vi "Project XML Editor.vi"() -> ()   [LabVIEW 2018, in ".LVLIBP CD XML Updater.lvlib" / "Project XML Editor.lvclass"]
uses:
  Project XML Editor.lvclass
  TypeDefs/Dependency Parameters.ctl
  Project XML Editor.lvclass/Project XML Editor.ctl
panel:
  out "XML Path":path
  out "Common Doc Dir":string
  out "CD Name":string
  out "Array":T1[](array[typedef])
  out "error out":errorcluster
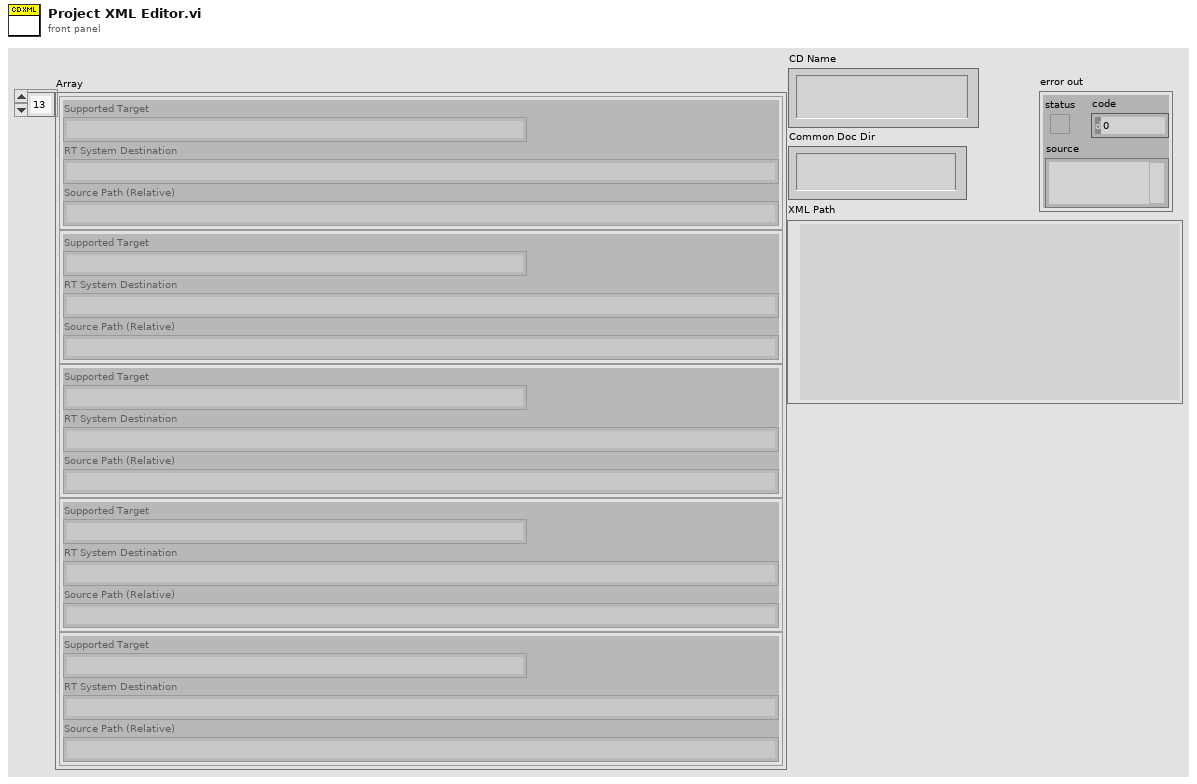
[diagram p1: front panel]
types:
  T1 = typedef ".LVLIBP CD XML Updater.lvlib/Project XML Editor.lvclass/Dependency Parameters.ctl" = cluster{"Supported Target":string, "RT System Destination":string, "Source Path (Relative)":string}
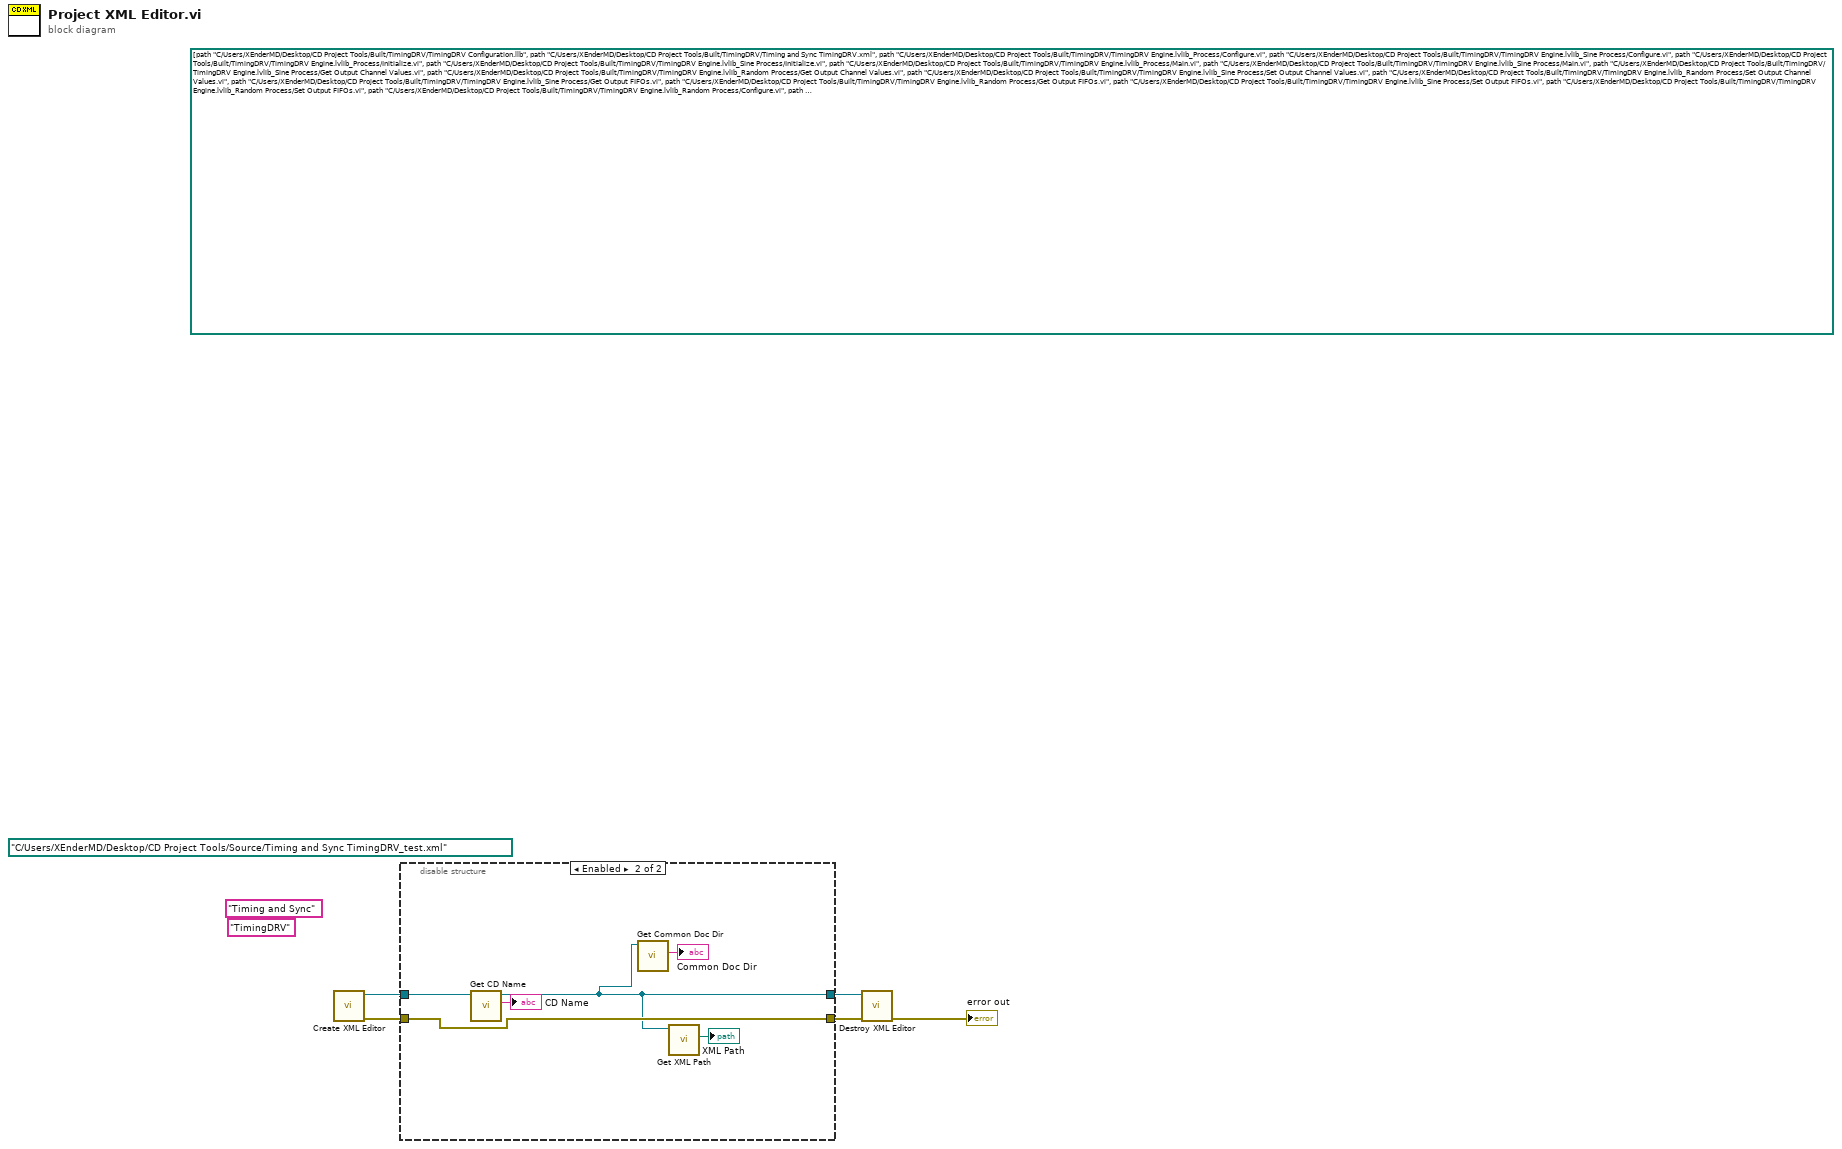
[diagram p0: block diagram]
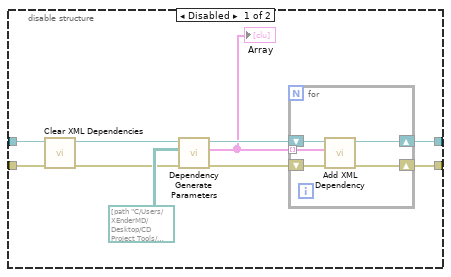
[diagram p2: hidden frame]
diagram:
  (unwired) "Timing and Sync" ("Common Doc Dir")
  (unwired) "TimingDRV" ("CD Name")
  (unwired) path "C:/Users/XEnderMD/Desktop/CD Project Tools/Source/Timing and Sync TimingDRV_test.xml" ("XML Path")
  (unwired) path[][] [[path "C:/Users/XEnderMD/Desktop/CD Project Tools/Built/TimingDRV/TimingDRV Configuration.llb", path "C:/Users/XEnderMD/Desktop/CD Project Tools/Built/TimingDRV/Timing and Sync TimingDRV.xml", path "C:/Users/XEnderMD/Desktop/CD Project Tools/Built/TimingDRV/TimingDRV Engine.lvlib_Process/Configure.vi", path "C:/Users/XEnderMD/Desktop/CD Project Tools/Built/TimingDRV/TimingDRV Engine.lvlib_Sine Process/Configure.vi", path "C:/Users/XEnderMD/Desktop/CD Project Tools/Built/TimingDRV/TimingDRV Engine.lvlib_Process/Initialize.vi", path "C:/Users/XEnderMD/Desktop/CD Project Tools/Built/TimingDRV/TimingDRV Engine.lvlib_Sine Process/Initialize.vi", path "C:/Users/XEnderMD/Desktop/CD Project Tools/Built/TimingDRV/TimingDRV Engine.lvlib_Process/Main.vi", path "C:/Users/XEnderMD/Desktop/CD Project Tools/Built/TimingDRV/TimingDRV Engine.lvlib_Sine Process/Main.vi", path "C:/Users/XEnderMD/Desktop/CD Project Tools/Built/TimingDRV/TimingDRV Engine.lvlib_Sine Process/Get Output Channel Values.vi", path "C:/Users/XEnderMD/Desktop/CD Project Tools/Built/TimingDRV/TimingDRV Engine.lvlib_Random Process/Get Output Channel Values.vi", path "C:/Users/XEnderMD/Desktop/CD Project Tools/Built/TimingDRV/TimingDRV Engine.lvlib_Sine Process/Set Output Channel Values.vi", path "C:/Users/XEnderMD/Desktop/CD Project Tools/Built/TimingDRV/TimingDRV Engine.lvlib_Random Process/Set Output Channel Values.vi", path "C:/Users/XEnderMD/Desktop/CD Project Tools/Built/TimingDRV/TimingDRV Engine.lvlib_Sine Process/Get Output FIFOs.vi", path "C:/Users/XEnderMD/Desktop/CD Project Tools/Built/TimingDRV/TimingDRV Engine.lvlib_Random Process/Get Output FIFOs.vi", path "C:/Users/XEnderMD/Desktop/CD Project Tools/Built/TimingDRV/TimingDRV Engine.lvlib_Sine Process/Set Output FIFOs.vi", path "C:/Users/XEnderMD/Desktop/CD Project Tools/Built/TimingDRV/TimingDRV Engine.lvlib_Random Process/Set Output FIFOs.vi", path "C:/Users/XEnderMD/Desktop/CD Project Tools/Built/TimingDRV/TimingDRV Engine.lvlib_Random Process/Configure.vi", path "C:/Users/XEnderMD/Desktop/CD Project Tools/Built/TimingDRV/TimingDRV Engine.lvlib_Random Process/Initialize.vi", path "C:/Users/XEnderMD/Desktop/CD Project Tools/Built/TimingDRV/TimingDRV Engine.lvlib_Sine Process/Initialize Output Channel Values.vi", path "C:/Users/XEnderMD/Desktop/CD Project Tools/Built/TimingDRV/TimingDRV Engine.lvlib_Random Process/Initialize Output Channel Values.vi", path "C:/Users/XEnderMD/Desktop/CD Project Tools/Built/TimingDRV/TimingDRV Engine.lvlib_Random Process/Main.vi", path "C:/Users/XEnderMD/Desktop/CD Project Tools/Built/TimingDRV/TimingDRV Engine.lvlib_Sine Process/Update Channel Value.vi", path "C:/Users/XEnderMD/Desktop/CD Project Tools/Built/TimingDRV/TimingDRV Engine.lvlib_Random Process/Update Channel Value.vi", path "", path "", path "", path "", path "", path "", path "", path "", path "", path "", path "", path "", path "", path "", path "", path "", path ""], [path "C:/Users/XEnderMD/Desktop/CD Project Tools/Built/TimingDRV/Windows/TimingDRV Engine Windows.llb", path "C:/Users/XEnderMD/Desktop/CD Project Tools/Built/TimingDRV/Windows/TimingDRV Engine.lvlib_Assembler/Main.vi", path "C:/Users/XEnderMD/Desktop/CD Project Tools/Built/TimingDRV/Windows/TimingDRV Engine.lvlib_Input Process/Main.vi", path "C:/Users/XEnderMD/Desktop/CD Project Tools/Built/TimingDRV/Windows/TimingDRV Engine.lvlib_Output Process/Initialize Output Channel Values.vi", path "C:/Users/XEnderMD/Desktop/CD Project Tools/Built/TimingDRV/Windows/TimingDRV Engine.lvlib_Sine Process/Initialize Output Channel Values.vi", path "C:/Users/XEnderMD/Desktop/CD Project Tools/Built/TimingDRV/Windows/TimingDRV Engine.lvlib_Output Process/Update Channel Value.vi", path "C:/Users/XEnderMD/Desktop/CD Project Tools/Built/TimingDRV/Windows/TimingDRV Engine.lvlib_Sine Process/Update Channel Value.vi", path "C:/Users/XEnderMD/Desktop/CD Project Tools/Built/TimingDRV/Windows/TimingDRV Engine.lvlib_Random Process/Initialize Output Channel Values.vi", path "C:/Users/XEnderMD/Desktop/CD Project Tools/Built/TimingDRV/Windows/TimingDRV Engine.lvlib_Random Process/Update Channel Value.vi", path "C:/Users/XEnderMD/Desktop/CD Project Tools/Built/TimingDRV/Windows/TimingDRV Engine.lvlib_Assembler/Configure.vi", path "C:/Users/XEnderMD/Desktop/CD Project Tools/Built/TimingDRV/Windows/TimingDRV Engine.lvlib_Output Process/Configure.vi", path "C:/Users/XEnderMD/Desktop/CD Project Tools/Built/TimingDRV/Windows/TimingDRV Engine.lvlib_Assembler/Initialize.vi", path "C:/Users/XEnderMD/Desktop/CD Project Tools/Built/TimingDRV/Windows/TimingDRV Engine.lvlib_Output Process/Initialize.vi", path "C:/Users/XEnderMD/Desktop/CD Project Tools/Built/TimingDRV/Windows/TimingDRV Engine.lvlib_Output Process/Main.vi", path "C:/Users/XEnderMD/Desktop/CD Project Tools/Built/TimingDRV/Windows/TimingDRV Engine.lvlib_Output Process/Get Output Channel Values.vi", path "C:/Users/XEnderMD/Desktop/CD Project Tools/Built/TimingDRV/Windows/TimingDRV Engine.lvlib_Sine Process/Get Output Channel Values.vi", path "C:/Users/XEnderMD/Desktop/CD Project Tools/Built/TimingDRV/Windows/TimingDRV Engine.lvlib_Output Process/Set Output Channel Values.vi", path "C:/Users/XEnderMD/Desktop/CD Project Tools/Built/TimingDRV/Windows/TimingDRV Engine.lvlib_Sine Process/Set Output Channel Values.vi", path "C:/Users/XEnderMD/Desktop/CD Project Tools/Built/TimingDRV/Windows/TimingDRV Engine.lvlib_Output Process/Get Output FIFOs.vi", path "C:/Users/XEnderMD/Desktop/CD Project Tools/Built/TimingDRV/Windows/TimingDRV Engine.lvlib_Sine Process/Get Output FIFOs.vi", path "C:/Users/XEnderMD/Desktop/CD Project Tools/Built/TimingDRV/Windows/TimingDRV Engine.lvlib_Output Process/Set Output FIFOs.vi", path "C:/Users/XEnderMD/Desktop/CD Project Tools/Built/TimingDRV/Windows/TimingDRV Engine.lvlib_Sine Process/Set Output FIFOs.vi", path "C:/Users/XEnderMD/Desktop/CD Project Tools/Built/TimingDRV/Windows/TimingDRV Engine.lvlib_Sine Process/Configure.vi", path "C:/Users/XEnderMD/Desktop/CD Project Tools/Built/TimingDRV/Windows/TimingDRV Engine.lvlib_Sine Process/Initialize.vi", path "C:/Users/XEnderMD/Desktop/CD Project Tools/Built/TimingDRV/Windows/TimingDRV Engine.lvlib_Sine Process/Main.vi", path "C:/Users/XEnderMD/Desktop/CD Project Tools/Built/TimingDRV/Windows/TimingDRV Engine.lvlib_Random Process/Get Output Channel Values.vi", path "C:/Users/XEnderMD/Desktop/CD Project Tools/Built/TimingDRV/Windows/TimingDRV Engine.lvlib_Random Process/Set Output Channel Values.vi", path "C:/Users/XEnderMD/Desktop/CD Project Tools/Built/TimingDRV/Windows/TimingDRV Engine.lvlib_Random Process/Get Output FIFOs.vi", path "C:/Users/XEnderMD/Desktop/CD Project Tools/Built/TimingDRV/Windows/TimingDRV Engine.lvlib_Random Process/Set Output FIFOs.vi", path "C:/Users/XEnderMD/Desktop/CD Project Tools/Built/TimingDRV/Windows/TimingDRV Engine.lvlib_Random Process/Configure.vi", path "C:/Users/XEnderMD/Desktop/CD Project Tools/Built/TimingDRV/Windows/TimingDRV Engine.lvlib_Random Process/Initialize.vi", path "C:/Users/XEnderMD/Desktop/CD Project Tools/Built/TimingDRV/Windows/TimingDRV Engine.lvlib_Random Process/Main.vi", path "C:/Users/XEnderMD/Desktop/CD Project Tools/Built/TimingDRV/Windows/TimingDRV Engine.lvlib_Process/Configure.vi", path "C:/Users/XEnderMD/Desktop/CD Project Tools/Built/TimingDRV/Windows/TimingDRV Engine.lvlib_Assembler/Launcher.vi", path "C:/Users/XEnderMD/Desktop/CD Project Tools/Built/TimingDRV/Windows/TimingDRV Engine.lvlib_Process/Launcher.vi", path "C:/Users/XEnderMD/Desktop/CD Project Tools/Built/TimingDRV/Windows/TimingDRV Engine.lvlib_Process/Initialize.vi", path "C:/Users/XEnderMD/Desktop/CD Project Tools/Built/TimingDRV/Windows/TimingDRV Engine.lvlib_Process/Main.vi", path "C:/Users/XEnderMD/Desktop/CD Project Tools/Built/TimingDRV/Windows/TimingDRV Engine.lvlib_Assembler/Shutdown.vi", path "C:/Users/XEnderMD/Desktop/CD Project Tools/Built/TimingDRV/Windows/TimingDRV Engine.lvlib_Process/Shutdown.vi", path ""], [path "C:/Users/XEnderMD/Desktop/CD Project Tools/Built/TimingDRV/Pharlap/TimingDRV Engine Pharlap.llb", path "C:/Users/XEnderMD/Desktop/CD Project Tools/Built/TimingDRV/Pharlap/TimingDRV Engine.lvlib_Assembler/Main.vi", path "C:/Users/XEnderMD/Desktop/CD Project Tools/Built/TimingDRV/Pharlap/TimingDRV Engine.lvlib_Input Process/Main.vi", path "C:/Users/XEnderMD/Desktop/CD Project Tools/Built/TimingDRV/Pharlap/TimingDRV Engine.lvlib_Output Process/Initialize Output Channel Values.vi", path "C:/Users/XEnderMD/Desktop/CD Project Tools/Built/TimingDRV/Pharlap/TimingDRV Engine.lvlib_Sine Process/Initialize Output Channel Values.vi", path "C:/Users/XEnderMD/Desktop/CD Project Tools/Built/TimingDRV/Pharlap/TimingDRV Engine.lvlib_Output Process/Update Channel Value.vi", path "C:/Users/XEnderMD/Desktop/CD Project Tools/Built/TimingDRV/Pharlap/TimingDRV Engine.lvlib_Sine Process/Update Channel Value.vi", path "C:/Users/XEnderMD/Desktop/CD Project Tools/Built/TimingDRV/Pharlap/TimingDRV Engine.lvlib_Random Process/Initialize Output Channel Values.vi", path "C:/Users/XEnderMD/Desktop/CD Project Tools/Built/TimingDRV/Pharlap/TimingDRV Engine.lvlib_Random Process/Update Channel Value.vi", path "C:/Users/XEnderMD/Desktop/CD Project Tools/Built/TimingDRV/Pharlap/TimingDRV Engine.lvlib_Assembler/Configure.vi", path "C:/Users/XEnderMD/Desktop/CD Project Tools/Built/TimingDRV/Pharlap/TimingDRV Engine.lvlib_Output Process/Configure.vi", path "C:/Users/XEnderMD/Desktop/CD Project Tools/Built/TimingDRV/Pharlap/TimingDRV Engine.lvlib_Assembler/Initialize.vi", path "C:/Users/XEnderMD/Desktop/CD Project Tools/Built/TimingDRV/Pharlap/TimingDRV Engine.lvlib_Output Process/Initialize.vi", path "C:/Users/XEnderMD/Desktop/CD Project Tools/Built/TimingDRV/Pharlap/TimingDRV Engine.lvlib_Output Process/Main.vi", path "C:/Users/XEnderMD/Desktop/CD Project Tools/Built/TimingDRV/Pharlap/TimingDRV Engine.lvlib_Output Process/Get Output Channel Values.vi", path "C:/Users/XEnderMD/Desktop/CD Project Tools/Built/TimingDRV/Pharlap/TimingDRV Engine.lvlib_Sine Process/Get Output Channel Values.vi", path "C:/Users/XEnderMD/Desktop/CD Project Tools/Built/TimingDRV/Pharlap/TimingDRV Engine.lvlib_Output Process/Set Output Channel Values.vi", path "C:/Users/XEnderMD/Desktop/CD Project Tools/Built/TimingDRV/Pharlap/TimingDRV Engine.lvlib_Sine Process/Set Output Channel Values.vi", path "C:/Users/XEnderMD/Desktop/CD Project Tools/Built/TimingDRV/Pharlap/TimingDRV Engine.lvlib_Output Process/Get Output FIFOs.vi", path "C:/Users/XEnderMD/Desktop/CD Project Tools/Built/TimingDRV/Pharlap/TimingDRV Engine.lvlib_Sine Process/Get Output FIFOs.vi", path "C:/Users/XEnderMD/Desktop/CD Project Tools/Built/TimingDRV/Pharlap/TimingDRV Engine.lvlib_Output Process/Set Output FIFOs.vi", path "C:/Users/XEnderMD/Desktop/CD Project Tools/Built/TimingDRV/Pharlap/TimingDRV Engine.lvlib_Sine Process/Set Output FIFOs.vi", path "C:/Users/XEnderMD/Desktop/CD Project Tools/Built/TimingDRV/Pharlap/TimingDRV Engine.lvlib_Sine Process/Configure.vi", path "C:/Users/XEnderMD/Desktop/CD Project Tools/Built/TimingDRV/Pharlap/TimingDRV Engine.lvlib_Sine Process/Initialize.vi", path "C:/Users/XEnderMD/Desktop/CD Project Tools/Built/TimingDRV/Pharlap/TimingDRV Engine.lvlib_Sine Process/Main.vi", path "C:/Users/XEnderMD/Desktop/CD Project Tools/Built/TimingDRV/Pharlap/TimingDRV Engine.lvlib_Random Process/Get Output Channel Values.vi", path "C:/Users/XEnderMD/Desktop/CD Project Tools/Built/TimingDRV/Pharlap/TimingDRV Engine.lvlib_Random Process/Set Output Channel Values.vi", path "C:/Users/XEnderMD/Desktop/CD Project Tools/Built/TimingDRV/Pharlap/TimingDRV Engine.lvlib_Random Process/Get Output FIFOs.vi", path "C:/Users/XEnderMD/Desktop/CD Project Tools/Built/TimingDRV/Pharlap/TimingDRV Engine.lvlib_Random Process/Set Output FIFOs.vi", path "C:/Users/XEnderMD/Desktop/CD Project Tools/Built/TimingDRV/Pharlap/TimingDRV Engine.lvlib_Random Process/Configure.vi", path "C:/Users/XEnderMD/Desktop/CD Project Tools/Built/TimingDRV/Pharlap/TimingDRV Engine.lvlib_Random Process/Initialize.vi", path "C:/Users/XEnderMD/Desktop/CD Project Tools/Built/TimingDRV/Pharlap/TimingDRV Engine.lvlib_Random Process/Main.vi", path "C:/Users/XEnderMD/Desktop/CD Project Tools/Built/TimingDRV/Pharlap/TimingDRV Engine.lvlib_Process/Configure.vi", path "C:/Users/XEnderMD/Desktop/CD Project Tools/Built/TimingDRV/Pharlap/TimingDRV Engine.lvlib_Assembler/Launcher.vi", path "C:/Users/XEnderMD/Desktop/CD Project Tools/Built/TimingDRV/Pharlap/TimingDRV Engine.lvlib_Process/Launcher.vi", path "C:/Users/XEnderMD/Desktop/CD Project Tools/Built/TimingDRV/Pharlap/TimingDRV Engine.lvlib_Process/Initialize.vi", path "C:/Users/XEnderMD/Desktop/CD Project Tools/Built/TimingDRV/Pharlap/TimingDRV Engine.lvlib_Process/Main.vi", path "C:/Users/XEnderMD/Desktop/CD Project Tools/Built/TimingDRV/Pharlap/TimingDRV Engine.lvlib_Assembler/Shutdown.vi", path "C:/Users/XEnderMD/Desktop/CD Project Tools/Built/TimingDRV/Pharlap/TimingDRV Engine.lvlib_Process/Shutdown.vi", path "C:/Users/XEnderMD/Desktop/CD Project Tools/Built/TimingDRV/Engine Release_depinstr.bin"], [path "C:/Users/XEnderMD/Desktop/CD Project Tools/Built/TimingDRV/VxWorks/TimingDRV Engine VxWorks.llb", path "C:/Users/XEnderMD/Desktop/CD Project Tools/Built/TimingDRV/VxWorks/TimingDRV Engine.lvlib_Assembler/Main.vi", path "C:/Users/XEnderMD/Desktop/CD Project Tools/Built/TimingDRV/VxWorks/TimingDRV Engine.lvlib_Input Process/Main.vi", path "C:/Users/XEnderMD/Desktop/CD Project Tools/Built/TimingDRV/VxWorks/TimingDRV Engine.lvlib_Output Process/Initialize Output Channel Values.vi", path "C:/Users/XEnderMD/Desktop/CD Project Tools/Built/TimingDRV/VxWorks/TimingDRV Engine.lvlib_Sine Process/Initialize Output Channel Values.vi", path "C:/Users/XEnderMD/Desktop/CD Project Tools/Built/TimingDRV/VxWorks/TimingDRV Engine.lvlib_Output Process/Update Channel Value.vi", path "C:/Users/XEnderMD/Desktop/CD Project Tools/Built/TimingDRV/VxWorks/TimingDRV Engine.lvlib_Sine Process/Update Channel Value.vi", path "C:/Users/XEnderMD/Desktop/CD Project Tools/Built/TimingDRV/VxWorks/TimingDRV Engine.lvlib_Random Process/Initialize Output Channel Values.vi", path "C:/Users/XEnderMD/Desktop/CD Project Tools/Built/TimingDRV/VxWorks/TimingDRV Engine.lvlib_Random Process/Update Channel Value.vi", path "C:/Users/XEnderMD/Desktop/CD Project Tools/Built/TimingDRV/VxWorks/TimingDRV Engine.lvlib_Assembler/Configure.vi", path "C:/Users/XEnderMD/Desktop/CD Project Tools/Built/TimingDRV/VxWorks/TimingDRV Engine.lvlib_Output Process/Configure.vi", path "C:/Users/XEnderMD/Desktop/CD Project Tools/Built/TimingDRV/VxWorks/TimingDRV Engine.lvlib_Assembler/Initialize.vi", path "C:/Users/XEnderMD/Desktop/CD Project Tools/Built/TimingDRV/VxWorks/TimingDRV Engine.lvlib_Output Process/Initialize.vi", path "C:/Users/XEnderMD/Desktop/CD Project Tools/Built/TimingDRV/VxWorks/TimingDRV Engine.lvlib_Output Process/Main.vi", path "C:/Users/XEnderMD/Desktop/CD Project Tools/Built/TimingDRV/VxWorks/TimingDRV Engine.lvlib_Output Process/Get Output Channel Values.vi", path "C:/Users/XEnderMD/Desktop/CD Project Tools/Built/TimingDRV/VxWorks/TimingDRV Engine.lvlib_Sine Process/Get Output Channel Values.vi", path "C:/Users/XEnderMD/Desktop/CD Project Tools/Built/TimingDRV/VxWorks/TimingDRV Engine.lvlib_Output Process/Set Output Channel Values.vi", path "C:/Users/XEnderMD/Desktop/CD Project Tools/Built/TimingDRV/VxWorks/TimingDRV Engine.lvlib_Sine Process/Set Output Channel Values.vi", path "C:/Users/XEnderMD/Desktop/CD Project Tools/Built/TimingDRV/VxWorks/TimingDRV Engine.lvlib_Output Process/Get Output FIFOs.vi", path "C:/Users/XEnderMD/Desktop/CD Project Tools/Built/TimingDRV/VxWorks/TimingDRV Engine.lvlib_Sine Process/Get Output FIFOs.vi", path "C:/Users/XEnderMD/Desktop/CD Project Tools/Built/TimingDRV/VxWorks/TimingDRV Engine.lvlib_Output Process/Set Output FIFOs.vi", path "C:/Users/XEnderMD/Desktop/CD Project Tools/Built/TimingDRV/VxWorks/TimingDRV Engine.lvlib_Sine Process/Set Output FIFOs.vi", path "C:/Users/XEnderMD/Desktop/CD Project Tools/Built/TimingDRV/VxWorks/TimingDRV Engine.lvlib_Sine Process/Configure.vi", path "C:/Users/XEnderMD/Desktop/CD Project Tools/Built/TimingDRV/VxWorks/TimingDRV Engine.lvlib_Sine Process/Initialize.vi", path "C:/Users/XEnderMD/Desktop/CD Project Tools/Built/TimingDRV/VxWorks/TimingDRV Engine.lvlib_Sine Process/Main.vi", path "C:/Users/XEnderMD/Desktop/CD Project Tools/Built/TimingDRV/VxWorks/TimingDRV Engine.lvlib_Random Process/Get Output Channel Values.vi", path "C:/Users/XEnderMD/Desktop/CD Project Tools/Built/TimingDRV/VxWorks/TimingDRV Engine.lvlib_Random Process/Set Output Channel Values.vi", path "C:/Users/XEnderMD/Desktop/CD Project Tools/Built/TimingDRV/VxWorks/TimingDRV Engine.lvlib_Random Process/Get Output FIFOs.vi", path "C:/Users/XEnderMD/Desktop/CD Project Tools/Built/TimingDRV/VxWorks/TimingDRV Engine.lvlib_Random Process/Set Output FIFOs.vi", path "C:/Users/XEnderMD/Desktop/CD Project Tools/Built/TimingDRV/VxWorks/TimingDRV Engine.lvlib_Random Process/Configure.vi", path "C:/Users/XEnderMD/Desktop/CD Project Tools/Built/TimingDRV/VxWorks/TimingDRV Engine.lvlib_Random Process/Initialize.vi", path "C:/Users/XEnderMD/Desktop/CD Project Tools/Built/TimingDRV/VxWorks/TimingDRV Engine.lvlib_Random Process/Main.vi", path "C:/Users/XEnderMD/Desktop/CD Project Tools/Built/TimingDRV/VxWorks/TimingDRV Engine.lvlib_Process/Configure.vi", path "C:/Users/XEnderMD/Desktop/CD Project Tools/Built/TimingDRV/VxWorks/TimingDRV Engine.lvlib_Assembler/Launcher.vi", path "C:/Users/XEnderMD/Desktop/CD Project Tools/Built/TimingDRV/VxWorks/TimingDRV Engine.lvlib_Process/Launcher.vi", path "C:/Users/XEnderMD/Desktop/CD Project Tools/Built/TimingDRV/VxWorks/TimingDRV Engine.lvlib_Process/Initialize.vi", path "C:/Users/XEnderMD/Desktop/CD Project Tools/Built/TimingDRV/VxWorks/TimingDRV Engine.lvlib_Process/Main.vi", path "C:/Users/XEnderMD/Desktop/CD Project Tools/Built/TimingDRV/VxWorks/TimingDRV Engine.lvlib_Assembler/Shutdown.vi", path "C:/Users/XEnderMD/Desktop/CD Project Tools/Built/TimingDRV/VxWorks/TimingDRV Engine.lvlib_Process/Shutdown.vi", path "C:/Users/XEnderMD/Desktop/CD Project Tools/Built/TimingDRV/Engine Release_depinstr.bin"], [path "C:/Users/XEnderMD/Desktop/CD Project Tools/Built/TimingDRV/Linux_32_ARM/TimingDRV Engine LinuxARM.llb", path "C:/Users/XEnderMD/Desktop/CD Project Tools/Built/TimingDRV/Linux_32_ARM/TimingDRV Engine.lvlib_Assembler/Main.vi", path "C:/Users/XEnderMD/Desktop/CD Project Tools/Built/TimingDRV/Linux_32_ARM/TimingDRV Engine.lvlib_Input Process/Main.vi", path "C:/Users/XEnderMD/Desktop/CD Project Tools/Built/TimingDRV/Linux_32_ARM/TimingDRV Engine.lvlib_Output Process/Initialize Output Channel Values.vi", path "C:/Users/XEnderMD/Desktop/CD Project Tools/Built/TimingDRV/Linux_32_ARM/TimingDRV Engine.lvlib_Sine Process/Initialize Output Channel Values.vi", path "C:/Users/XEnderMD/Desktop/CD Project Tools/Built/TimingDRV/Linux_32_ARM/TimingDRV Engine.lvlib_Output Process/Update Channel Value.vi", path "C:/Users/XEnderMD/Desktop/CD Project Tools/Built/TimingDRV/Linux_32_ARM/TimingDRV Engine.lvlib_Sine Process/Update Channel Value.vi", path "C:/Users/XEnderMD/Desktop/CD Project Tools/Built/TimingDRV/Linux_32_ARM/TimingDRV Engine.lvlib_Random Process/Initialize Output Channel Values.vi", path "C:/Users/XEnderMD/Desktop/CD Project Tools/Built/TimingDRV/Linux_32_ARM/TimingDRV Engine.lvlib_Random Process/Update Channel Value.vi", path "C:/Users/XEnderMD/Desktop/CD Project Tools/Built/TimingDRV/Linux_32_ARM/TimingDRV Engine.lvlib_Assembler/Configure.vi", path "C:/Users/XEnderMD/Desktop/CD Project Tools/Built/TimingDRV/Linux_32_ARM/TimingDRV Engine.lvlib_Output Process/Configure.vi", path "C:/Users/XEnderMD/Desktop/CD Project Tools/Built/TimingDRV/Linux_32_ARM/TimingDRV Engine.lvlib_Assembler/Initialize.vi", path "C:/Users/XEnderMD/Desktop/CD Project Tools/Built/TimingDRV/Linux_32_ARM/TimingDRV Engine.lvlib_Output Process/Initialize.vi", path "C:/Users/XEnderMD/Desktop/CD Project Tools/Built/TimingDRV/Linux_32_ARM/TimingDRV Engine.lvlib_Output Process/Main.vi", path "C:/Users/XEnderMD/Desktop/CD Project Tools/Built/TimingDRV/Linux_32_ARM/TimingDRV Engine.lvlib_Output Process/Get Output Channel Values.vi", path "C:/Users/XEnderMD/Desktop/CD Project Tools/Built/TimingDRV/Linux_32_ARM/TimingDRV Engine.lvlib_Sine Process/Get Output Channel Values.vi", path "C:/Users/XEnderMD/Desktop/CD Project Tools/Built/TimingDRV/Linux_32_ARM/TimingDRV Engine.lvlib_Output Process/Set Output Channel Values.vi", path "C:/Users/XEnderMD/Desktop/CD Project Tools/Built/TimingDRV/Linux_32_ARM/TimingDRV Engine.lvlib_Sine Process/Set Output Channel Values.vi", path "C:/Users/XEnderMD/Desktop/CD Project Tools/Built/TimingDRV/Linux_32_ARM/TimingDRV Engine.lvlib_Output Process/Get Output FIFOs.vi", path "C:/Users/XEnderMD/Desktop/CD Project Tools/Built/TimingDRV/Linux_32_ARM/TimingDRV Engine.lvlib_Sine Process/Get Output FIFOs.vi", path "C:/Users/XEnderMD/Desktop/CD Project Tools/Built/TimingDRV/Linux_32_ARM/TimingDRV Engine.lvlib_Output Process/Set Output FIFOs.vi", path "C:/Users/XEnderMD/Desktop/CD Project Tools/Built/TimingDRV/Linux_32_ARM/TimingDRV Engine.lvlib_Sine Process/Set Output FIFOs.vi", path "C:/Users/XEnderMD/Desktop/CD Project Tools/Built/TimingDRV/Linux_32_ARM/TimingDRV Engine.lvlib_Sine Process/Configure.vi", path "C:/Users/XEnderMD/Desktop/CD Project Tools/Built/TimingDRV/Linux_32_ARM/TimingDRV Engine.lvlib_Sine Process/Initialize.vi", path "C:/Users/XEnderMD/Desktop/CD Project Tools/Built/TimingDRV/Linux_32_ARM/TimingDRV Engine.lvlib_Sine Process/Main.vi", path "C:/Users/XEnderMD/Desktop/CD Project Tools/Built/TimingDRV/Linux_32_ARM/TimingDRV Engine.lvlib_Random Process/Get Output Channel Values.vi", path "C:/Users/XEnderMD/Desktop/CD Project Tools/Built/TimingDRV/Linux_32_ARM/TimingDRV Engine.lvlib_Random Process/Set Output Channel Values.vi", path "C:/Users/XEnderMD/Desktop/CD Project Tools/Built/TimingDRV/Linux_32_ARM/TimingDRV Engine.lvlib_Random Process/Get Output FIFOs.vi", path "C:/Users/XEnderMD/Desktop/CD Project Tools/Built/TimingDRV/Linux_32_ARM/TimingDRV Engine.lvlib_Random Process/Set Output FIFOs.vi", path "C:/Users/XEnderMD/Desktop/CD Project Tools/Built/TimingDRV/Linux_32_ARM/TimingDRV Engine.lvlib_Random Process/Configure.vi", path "C:/Users/XEnderMD/Desktop/CD Project Tools/Built/TimingDRV/Linux_32_ARM/TimingDRV Engine.lvlib_Random Process/Initialize.vi", path "C:/Users/XEnderMD/Desktop/CD Project Tools/Built/TimingDRV/Linux_32_ARM/TimingDRV Engine.lvlib_Random Process/Main.vi", path "C:/Users/XEnderMD/Desktop/CD Project Tools/Built/TimingDRV/Linux_32_ARM/TimingDRV Engine.lvlib_Process/Configure.vi", path "C:/Users/XEnderMD/Desktop/CD Project Tools/Built/TimingDRV/Linux_32_ARM/TimingDRV Engine.lvlib_Assembler/Launcher.vi", path "C:/Users/XEnderMD/Desktop/CD Project Tools/Built/TimingDRV/Linux_32_ARM/TimingDRV Engine.lvlib_Process/Launcher.vi", path "C:/Users/XEnderMD/Desktop/CD Project Tools/Built/TimingDRV/Linux_32_ARM/TimingDRV Engine.lvlib_Process/Initialize.vi", path "C:/Users/XEnderMD/Desktop/CD Project Tools/Built/TimingDRV/Linux_32_ARM/TimingDRV Engine.lvlib_Process/Main.vi", path "C:/Users/XEnderMD/Desktop/CD Project Tools/Built/TimingDRV/Linux_32_ARM/TimingDRV Engine.lvlib_Assembler/Shutdown.vi", path "C:/Users/XEnderMD/Desktop/CD Project Tools/Built/TimingDRV/Linux_32_ARM/TimingDRV Engine.lvlib_Process/Shutdown.vi", path "C:/Users/XEnderMD/Desktop/CD Project Tools/Built/TimingDRV/Engine Release_depinstr.bin"], [path "C:/Users/XEnderMD/Desktop/CD Project Tools/Built/TimingDRV/Linux_x64/TimingDRV Engine Linux64.llb", path "C:/Users/XEnderMD/Desktop/CD Project Tools/Built/TimingDRV/Linux_x64/TimingDRV Engine.lvlib_Assembler/Main.vi", path "C:/Users/XEnderMD/Desktop/CD Project Tools/Built/TimingDRV/Linux_x64/TimingDRV Engine.lvlib_Input Process/Main.vi", path "C:/Users/XEnderMD/Desktop/CD Project Tools/Built/TimingDRV/Linux_x64/TimingDRV Engine.lvlib_Output Process/Initialize Output Channel Values.vi", path "C:/Users/XEnderMD/Desktop/CD Project Tools/Built/TimingDRV/Linux_x64/TimingDRV Engine.lvlib_Sine Process/Initialize Output Channel Values.vi", path "C:/Users/XEnderMD/Desktop/CD Project Tools/Built/TimingDRV/Linux_x64/TimingDRV Engine.lvlib_Output Process/Update Channel Value.vi", path "C:/Users/XEnderMD/Desktop/CD Project Tools/Built/TimingDRV/Linux_x64/TimingDRV Engine.lvlib_Sine Process/Update Channel Value.vi", path "C:/Users/XEnderMD/Desktop/CD Project Tools/Built/TimingDRV/Linux_x64/TimingDRV Engine.lvlib_Random Process/Initialize Output Channel Values.vi", path "C:/Users/XEnderMD/Desktop/CD Project Tools/Built/TimingDRV/Linux_x64/TimingDRV Engine.lvlib_Random Process/Update Channel Value.vi", path "C:/Users/XEnderMD/Desktop/CD Project Tools/Built/TimingDRV/Linux_x64/TimingDRV Engine.lvlib_Assembler/Configure.vi", path "C:/Users/XEnderMD/Desktop/CD Project Tools/Built/TimingDRV/Linux_x64/TimingDRV Engine.lvlib_Output Process/Configure.vi", path "C:/Users/XEnderMD/Desktop/CD Project Tools/Built/TimingDRV/Linux_x64/TimingDRV Engine.lvlib_Assembler/Initialize.vi", path "C:/Users/XEnderMD/Desktop/CD Project Tools/Built/TimingDRV/Linux_x64/TimingDRV Engine.lvlib_Output Process/Initialize.vi", path "C:/Users/XEnderMD/Desktop/CD Project Tools/Built/TimingDRV/Linux_x64/TimingDRV Engine.lvlib_Output Process/Main.vi", path "C:/Users/XEnderMD/Desktop/CD Project Tools/Built/TimingDRV/Linux_x64/TimingDRV Engine.lvlib_Output Process/Get Output Channel Values.vi", path "C:/Users/XEnderMD/Desktop/CD Project Tools/Built/TimingDRV/Linux_x64/TimingDRV Engine.lvlib_Sine Process/Get Output Channel Values.vi", path "C:/Users/XEnderMD/Desktop/CD Project Tools/Built/TimingDRV/Linux_x64/TimingDRV Engine.lvlib_Output Process/Set Output Channel Values.vi", path "C:/Users/XEnderMD/Desktop/CD Project Tools/Built/TimingDRV/Linux_x64/TimingDRV Engine.lvlib_Sine Process/Set Output Channel Values.vi", path "C:/Users/XEnderMD/Desktop/CD Project Tools/Built/TimingDRV/Linux_x64/TimingDRV Engine.lvlib_Output Process/Get Output FIFOs.vi", path "C:/Users/XEnderMD/Desktop/CD Project Tools/Built/TimingDRV/Linux_x64/TimingDRV Engine.lvlib_Sine Process/Get Output FIFOs.vi", path "C:/Users/XEnderMD/Desktop/CD Project Tools/Built/TimingDRV/Linux_x64/TimingDRV Engine.lvlib_Output Process/Set Output FIFOs.vi", path "C:/Users/XEnderMD/Desktop/CD Project Tools/Built/TimingDRV/Linux_x64/TimingDRV Engine.lvlib_Sine Process/Set Output FIFOs.vi", path "C:/Users/XEnderMD/Desktop/CD Project Tools/Built/TimingDRV/Linux_x64/TimingDRV Engine.lvlib_Sine Process/Configure.vi", path "C:/Users/XEnderMD/Desktop/CD Project Tools/Built/TimingDRV/Linux_x64/TimingDRV Engine.lvlib_Sine Process/Initialize.vi", path "C:/Users/XEnderMD/Desktop/CD Project Tools/Built/TimingDRV/Linux_x64/TimingDRV Engine.lvlib_Sine Process/Main.vi", path "C:/Users/XEnderMD/Desktop/CD Project Tools/Built/TimingDRV/Linux_x64/TimingDRV Engine.lvlib_Random Process/Get Output Channel Values.vi", path "C:/Users/XEnderMD/Desktop/CD Project Tools/Built/TimingDRV/Linux_x64/TimingDRV Engine.lvlib_Random Process/Set Output Channel Values.vi", path "C:/Users/XEnderMD/Desktop/CD Project Tools/Built/TimingDRV/Linux_x64/TimingDRV Engine.lvlib_Random Process/Get Output FIFOs.vi", path "C:/Users/XEnderMD/Desktop/CD Project Tools/Built/TimingDRV/Linux_x64/TimingDRV Engine.lvlib_Random Process/Set Output FIFOs.vi", path "C:/Users/XEnderMD/Desktop/CD Project Tools/Built/TimingDRV/Linux_x64/TimingDRV Engine.lvlib_Random Process/Configure.vi", path "C:/Users/XEnderMD/Desktop/CD Project Tools/Built/TimingDRV/Linux_x64/TimingDRV Engine.lvlib_Random Process/Initialize.vi", path "C:/Users/XEnderMD/Desktop/CD Project Tools/Built/TimingDRV/Linux_x64/TimingDRV Engine.lvlib_Random Process/Main.vi", path "C:/Users/XEnderMD/Desktop/CD Project Tools/Built/TimingDRV/Linux_x64/TimingDRV Engine.lvlib_Process/Configure.vi", path "C:/Users/XEnderMD/Desktop/CD Project Tools/Built/TimingDRV/Linux_x64/TimingDRV Engine.lvlib_Assembler/Launcher.vi", path "C:/Users/XEnderMD/Desktop/CD Project Tools/Built/TimingDRV/Linux_x64/TimingDRV Engine.lvlib_Process/Launcher.vi", path "C:/Users/XEnderMD/Desktop/CD Project Tools/Built/TimingDRV/Linux_x64/TimingDRV Engine.lvlib_Process/Initialize.vi", path "C:/Users/XEnderMD/Desktop/CD Project Tools/Built/TimingDRV/Linux_x64/TimingDRV Engine.lvlib_Process/Main.vi", path "C:/Users/XEnderMD/Desktop/CD Project Tools/Built/TimingDRV/Linux_x64/TimingDRV Engine.lvlib_Assembler/Shutdown.vi", path "C:/Users/XEnderMD/Desktop/CD Project Tools/Built/TimingDRV/Linux_x64/TimingDRV Engine.lvlib_Process/Shutdown.vi", path "C:/Users/XEnderMD/Desktop/CD Project Tools/Built/TimingDRV/Engine Release_depinstr.bin"]] ("Generated files 2")
  n1 = call "Create XML Editor.vi"() -> ("error out"=w1:errorcluster, "Project XML Editor out"=w2:refnum<class "Project XML Editor.lvclass">)  [unwired: 10 in]
  n2 = disable-structure shown="Enabled" {
    disable-tunnel: [w14 w22] -> w4
    disable-tunnel: [w13 w25] -> w3
    disable-tunnel: w2 -> [w12 w26]
    disable-tunnel: w1 -> [w11 w25]
    frame Disabled {
      n3 = call "Clear XML Dependencies.vi"("error in (no error)"=w11, "Project XML Editor in"=w12) -> ("error out"=w10:errorcluster, "Project XML Editor out"=w9:refnum<class "Project XML Editor.lvclass">)  [unwired: 8 in]
      n4 = call "Dependency Generate Parameters.vi"("error in (no error)"=w10, "Generated files in"=path[][] [[path "C:/Users/XEnderMD/Desktop/CD Project Tools/Built/TimingDRV/TimingDRV Configuration.llb", path "C:/Users/XEnderMD/Desktop/CD Project Tools/Built/TimingDRV/Timing and Sync TimingDRV.xml", path "C:/Users/XEnderMD/Desktop/CD Project Tools/Built/TimingDRV/TimingDRV Engine.lvlib_Process/Configure.vi", path "C:/Users/XEnderMD/Desktop/CD Project Tools/Built/TimingDRV/TimingDRV Engine.lvlib_Sine Process/Configure.vi", path "C:/Users/XEnderMD/Desktop/CD Project Tools/Built/TimingDRV/TimingDRV Engine.lvlib_Process/Initialize.vi", path "C:/Users/XEnderMD/Desktop/CD Project Tools/Built/TimingDRV/TimingDRV Engine.lvlib_Sine Process/Initialize.vi", path "C:/Users/XEnderMD/Desktop/CD Project Tools/Built/TimingDRV/TimingDRV Engine.lvlib_Process/Main.vi", path "C:/Users/XEnderMD/Desktop/CD Project Tools/Built/TimingDRV/TimingDRV Engine.lvlib_Sine Process/Main.vi", path "C:/Users/XEnderMD/Desktop/CD Project Tools/Built/TimingDRV/TimingDRV Engine.lvlib_Sine Process/Get Output Channel Values.vi", path "C:/Users/XEnderMD/Desktop/CD Project Tools/Built/TimingDRV/TimingDRV Engine.lvlib_Random Process/Get Output Channel Values.vi", path "C:/Users/XEnderMD/Desktop/CD Project Tools/Built/TimingDRV/TimingDRV Engine.lvlib_Sine Process/Set Output Channel Values.vi", path "C:/Users/XEnderMD/Desktop/CD Project Tools/Built/TimingDRV/TimingDRV Engine.lvlib_Random Process/Set Output Channel Values.vi", path "C:/Users/XEnderMD/Desktop/CD Project Tools/Built/TimingDRV/TimingDRV Engine.lvlib_Sine Process/Get Output FIFOs.vi", path "C:/Users/XEnderMD/Desktop/CD Project Tools/Built/TimingDRV/TimingDRV Engine.lvlib_Random Process/Get Output FIFOs.vi", path "C:/Users/XEnderMD/Desktop/CD Project Tools/Built/TimingDRV/TimingDRV Engine.lvlib_Sine Process/Set Output FIFOs.vi", path "C:/Users/XEnderMD/Desktop/CD Project Tools/Built/TimingDRV/TimingDRV Engine.lvlib_Random Process/Set Output FIFOs.vi", path "C:/Users/XEnderMD/Desktop/CD Project Tools/Built/TimingDRV/TimingDRV Engine.lvlib_Random Process/Configure.vi", path "C:/Users/XEnderMD/Desktop/CD Project Tools/Built/TimingDRV/TimingDRV Engine.lvlib_Random Process/Initialize.vi", path "C:/Users/XEnderMD/Desktop/CD Project Tools/Built/TimingDRV/TimingDRV Engine.lvlib_Sine Process/Initialize Output Channel Values.vi", path "C:/Users/XEnderMD/Desktop/CD Project Tools/Built/TimingDRV/TimingDRV Engine.lvlib_Random Process/Initialize Output Channel Values.vi", path "C:/Users/XEnderMD/Desktop/CD Project Tools/Built/TimingDRV/TimingDRV Engine.lvlib_Random Process/Main.vi", path "C:/Users/XEnderMD/Desktop/CD Project Tools/Built/TimingDRV/TimingDRV Engine.lvlib_Sine Process/Update Channel Value.vi", path "C:/Users/XEnderMD/Desktop/CD Project Tools/Built/TimingDRV/TimingDRV Engine.lvlib_Random Process/Update Channel Value.vi", path "", path "", path "", path "", path "", path "", path "", path "", path "", path "", path "", path "", path "", path "", path "", path "", path ""], [path "C:/Users/XEnderMD/Desktop/CD Project Tools/Built/TimingDRV/Windows/TimingDRV Engine Windows.llb", path "C:/Users/XEnderMD/Desktop/CD Project Tools/Built/TimingDRV/Windows/TimingDRV Engine.lvlib_Assembler/Main.vi", path "C:/Users/XEnderMD/Desktop/CD Project Tools/Built/TimingDRV/Windows/TimingDRV Engine.lvlib_Input Process/Main.vi", path "C:/Users/XEnderMD/Desktop/CD Project Tools/Built/TimingDRV/Windows/TimingDRV Engine.lvlib_Output Process/Initialize Output Channel Values.vi", path "C:/Users/XEnderMD/Desktop/CD Project Tools/Built/TimingDRV/Windows/TimingDRV Engine.lvlib_Sine Process/Initialize Output Channel Values.vi", path "C:/Users/XEnderMD/Desktop/CD Project Tools/Built/TimingDRV/Windows/TimingDRV Engine.lvlib_Output Process/Update Channel Value.vi", path "C:/Users/XEnderMD/Desktop/CD Project Tools/Built/TimingDRV/Windows/TimingDRV Engine.lvlib_Sine Process/Update Channel Value.vi", path "C:/Users/XEnderMD/Desktop/CD Project Tools/Built/TimingDRV/Windows/TimingDRV Engine.lvlib_Random Process/Initialize Output Channel Values.vi", path "C:/Users/XEnderMD/Desktop/CD Project Tools/Built/TimingDRV/Windows/TimingDRV Engine.lvlib_Random Process/Update Channel Value.vi", path "C:/Users/XEnderMD/Desktop/CD Project Tools/Built/TimingDRV/Windows/TimingDRV Engine.lvlib_Assembler/Configure.vi", path "C:/Users/XEnderMD/Desktop/CD Project Tools/Built/TimingDRV/Windows/TimingDRV Engine.lvlib_Output Process/Configure.vi", path "C:/Users/XEnderMD/Desktop/CD Project Tools/Built/TimingDRV/Windows/TimingDRV Engine.lvlib_Assembler/Initialize.vi", path "C:/Users/XEnderMD/Desktop/CD Project Tools/Built/TimingDRV/Windows/TimingDRV Engine.lvlib_Output Process/Initialize.vi", path "C:/Users/XEnderMD/Desktop/CD Project Tools/Built/TimingDRV/Windows/TimingDRV Engine.lvlib_Output Process/Main.vi", path "C:/Users/XEnderMD/Desktop/CD Project Tools/Built/TimingDRV/Windows/TimingDRV Engine.lvlib_Output Process/Get Output Channel Values.vi", path "C:/Users/XEnderMD/Desktop/CD Project Tools/Built/TimingDRV/Windows/TimingDRV Engine.lvlib_Sine Process/Get Output Channel Values.vi", path "C:/Users/XEnderMD/Desktop/CD Project Tools/Built/TimingDRV/Windows/TimingDRV Engine.lvlib_Output Process/Set Output Channel Values.vi", path "C:/Users/XEnderMD/Desktop/CD Project Tools/Built/TimingDRV/Windows/TimingDRV Engine.lvlib_Sine Process/Set Output Channel Values.vi", path "C:/Users/XEnderMD/Desktop/CD Project Tools/Built/TimingDRV/Windows/TimingDRV Engine.lvlib_Output Process/Get Output FIFOs.vi", path "C:/Users/XEnderMD/Desktop/CD Project Tools/Built/TimingDRV/Windows/TimingDRV Engine.lvlib_Sine Process/Get Output FIFOs.vi", path "C:/Users/XEnderMD/Desktop/CD Project Tools/Built/TimingDRV/Windows/TimingDRV Engine.lvlib_Output Process/Set Output FIFOs.vi", path "C:/Users/XEnderMD/Desktop/CD Project Tools/Built/TimingDRV/Windows/TimingDRV Engine.lvlib_Sine Process/Set Output FIFOs.vi", path "C:/Users/XEnderMD/Desktop/CD Project Tools/Built/TimingDRV/Windows/TimingDRV Engine.lvlib_Sine Process/Configure.vi", path "C:/Users/XEnderMD/Desktop/CD Project Tools/Built/TimingDRV/Windows/TimingDRV Engine.lvlib_Sine Process/Initialize.vi", path "C:/Users/XEnderMD/Desktop/CD Project Tools/Built/TimingDRV/Windows/TimingDRV Engine.lvlib_Sine Process/Main.vi", path "C:/Users/XEnderMD/Desktop/CD Project Tools/Built/TimingDRV/Windows/TimingDRV Engine.lvlib_Random Process/Get Output Channel Values.vi", path "C:/Users/XEnderMD/Desktop/CD Project Tools/Built/TimingDRV/Windows/TimingDRV Engine.lvlib_Random Process/Set Output Channel Values.vi", path "C:/Users/XEnderMD/Desktop/CD Project Tools/Built/TimingDRV/Windows/TimingDRV Engine.lvlib_Random Process/Get Output FIFOs.vi", path "C:/Users/XEnderMD/Desktop/CD Project Tools/Built/TimingDRV/Windows/TimingDRV Engine.lvlib_Random Process/Set Output FIFOs.vi", path "C:/Users/XEnderMD/Desktop/CD Project Tools/Built/TimingDRV/Windows/TimingDRV Engine.lvlib_Random Process/Configure.vi", path "C:/Users/XEnderMD/Desktop/CD Project Tools/Built/TimingDRV/Windows/TimingDRV Engine.lvlib_Random Process/Initialize.vi", path "C:/Users/XEnderMD/Desktop/CD Project Tools/Built/TimingDRV/Windows/TimingDRV Engine.lvlib_Random Process/Main.vi", path "C:/Users/XEnderMD/Desktop/CD Project Tools/Built/TimingDRV/Windows/TimingDRV Engine.lvlib_Process/Configure.vi", path "C:/Users/XEnderMD/Desktop/CD Project Tools/Built/TimingDRV/Windows/TimingDRV Engine.lvlib_Assembler/Launcher.vi", path "C:/Users/XEnderMD/Desktop/CD Project Tools/Built/TimingDRV/Windows/TimingDRV Engine.lvlib_Process/Launcher.vi", path "C:/Users/XEnderMD/Desktop/CD Project Tools/Built/TimingDRV/Windows/TimingDRV Engine.lvlib_Process/Initialize.vi", path "C:/Users/XEnderMD/Desktop/CD Project Tools/Built/TimingDRV/Windows/TimingDRV Engine.lvlib_Process/Main.vi", path "C:/Users/XEnderMD/Desktop/CD Project Tools/Built/TimingDRV/Windows/TimingDRV Engine.lvlib_Assembler/Shutdown.vi", path "C:/Users/XEnderMD/Desktop/CD Project Tools/Built/TimingDRV/Windows/TimingDRV Engine.lvlib_Process/Shutdown.vi", path ""], [path "C:/Users/XEnderMD/Desktop/CD Project Tools/Built/TimingDRV/Pharlap/TimingDRV Engine Pharlap.llb", path "C:/Users/XEnderMD/Desktop/CD Project Tools/Built/TimingDRV/Pharlap/TimingDRV Engine.lvlib_Assembler/Main.vi", path "C:/Users/XEnderMD/Desktop/CD Project Tools/Built/TimingDRV/Pharlap/TimingDRV Engine.lvlib_Input Process/Main.vi", path "C:/Users/XEnderMD/Desktop/CD Project Tools/Built/TimingDRV/Pharlap/TimingDRV Engine.lvlib_Output Process/Initialize Output Channel Values.vi", path "C:/Users/XEnderMD/Desktop/CD Project Tools/Built/TimingDRV/Pharlap/TimingDRV Engine.lvlib_Sine Process/Initialize Output Channel Values.vi", path "C:/Users/XEnderMD/Desktop/CD Project Tools/Built/TimingDRV/Pharlap/TimingDRV Engine.lvlib_Output Process/Update Channel Value.vi", path "C:/Users/XEnderMD/Desktop/CD Project Tools/Built/TimingDRV/Pharlap/TimingDRV Engine.lvlib_Sine Process/Update Channel Value.vi", path "C:/Users/XEnderMD/Desktop/CD Project Tools/Built/TimingDRV/Pharlap/TimingDRV Engine.lvlib_Random Process/Initialize Output Channel Values.vi", path "C:/Users/XEnderMD/Desktop/CD Project Tools/Built/TimingDRV/Pharlap/TimingDRV Engine.lvlib_Random Process/Update Channel Value.vi", path "C:/Users/XEnderMD/Desktop/CD Project Tools/Built/TimingDRV/Pharlap/TimingDRV Engine.lvlib_Assembler/Configure.vi", path "C:/Users/XEnderMD/Desktop/CD Project Tools/Built/TimingDRV/Pharlap/TimingDRV Engine.lvlib_Output Process/Configure.vi", path "C:/Users/XEnderMD/Desktop/CD Project Tools/Built/TimingDRV/Pharlap/TimingDRV Engine.lvlib_Assembler/Initialize.vi", path "C:/Users/XEnderMD/Desktop/CD Project Tools/Built/TimingDRV/Pharlap/TimingDRV Engine.lvlib_Output Process/Initialize.vi", path "C:/Users/XEnderMD/Desktop/CD Project Tools/Built/TimingDRV/Pharlap/TimingDRV Engine.lvlib_Output Process/Main.vi", path "C:/Users/XEnderMD/Desktop/CD Project Tools/Built/TimingDRV/Pharlap/TimingDRV Engine.lvlib_Output Process/Get Output Channel Values.vi", path "C:/Users/XEnderMD/Desktop/CD Project Tools/Built/TimingDRV/Pharlap/TimingDRV Engine.lvlib_Sine Process/Get Output Channel Values.vi", path "C:/Users/XEnderMD/Desktop/CD Project Tools/Built/TimingDRV/Pharlap/TimingDRV Engine.lvlib_Output Process/Set Output Channel Values.vi", path "C:/Users/XEnderMD/Desktop/CD Project Tools/Built/TimingDRV/Pharlap/TimingDRV Engine.lvlib_Sine Process/Set Output Channel Values.vi", path "C:/Users/XEnderMD/Desktop/CD Project Tools/Built/TimingDRV/Pharlap/TimingDRV Engine.lvlib_Output Process/Get Output FIFOs.vi", path "C:/Users/XEnderMD/Desktop/CD Project Tools/Built/TimingDRV/Pharlap/TimingDRV Engine.lvlib_Sine Process/Get Output FIFOs.vi", path "C:/Users/XEnderMD/Desktop/CD Project Tools/Built/TimingDRV/Pharlap/TimingDRV Engine.lvlib_Output Process/Set Output FIFOs.vi", path "C:/Users/XEnderMD/Desktop/CD Project Tools/Built/TimingDRV/Pharlap/TimingDRV Engine.lvlib_Sine Process/Set Output FIFOs.vi", path "C:/Users/XEnderMD/Desktop/CD Project Tools/Built/TimingDRV/Pharlap/TimingDRV Engine.lvlib_Sine Process/Configure.vi", path "C:/Users/XEnderMD/Desktop/CD Project Tools/Built/TimingDRV/Pharlap/TimingDRV Engine.lvlib_Sine Process/Initialize.vi", path "C:/Users/XEnderMD/Desktop/CD Project Tools/Built/TimingDRV/Pharlap/TimingDRV Engine.lvlib_Sine Process/Main.vi", path "C:/Users/XEnderMD/Desktop/CD Project Tools/Built/TimingDRV/Pharlap/TimingDRV Engine.lvlib_Random Process/Get Output Channel Values.vi", path "C:/Users/XEnderMD/Desktop/CD Project Tools/Built/TimingDRV/Pharlap/TimingDRV Engine.lvlib_Random Process/Set Output Channel Values.vi", path "C:/Users/XEnderMD/Desktop/CD Project Tools/Built/TimingDRV/Pharlap/TimingDRV Engine.lvlib_Random Process/Get Output FIFOs.vi", path "C:/Users/XEnderMD/Desktop/CD Project Tools/Built/TimingDRV/Pharlap/TimingDRV Engine.lvlib_Random Process/Set Output FIFOs.vi", path "C:/Users/XEnderMD/Desktop/CD Project Tools/Built/TimingDRV/Pharlap/TimingDRV Engine.lvlib_Random Process/Configure.vi", path "C:/Users/XEnderMD/Desktop/CD Project Tools/Built/TimingDRV/Pharlap/TimingDRV Engine.lvlib_Random Process/Initialize.vi", path "C:/Users/XEnderMD/Desktop/CD Project Tools/Built/TimingDRV/Pharlap/TimingDRV Engine.lvlib_Random Process/Main.vi", path "C:/Users/XEnderMD/Desktop/CD Project Tools/Built/TimingDRV/Pharlap/TimingDRV Engine.lvlib_Process/Configure.vi", path "C:/Users/XEnderMD/Desktop/CD Project Tools/Built/TimingDRV/Pharlap/TimingDRV Engine.lvlib_Assembler/Launcher.vi", path "C:/Users/XEnderMD/Desktop/CD Project Tools/Built/TimingDRV/Pharlap/TimingDRV Engine.lvlib_Process/Launcher.vi", path "C:/Users/XEnderMD/Desktop/CD Project Tools/Built/TimingDRV/Pharlap/TimingDRV Engine.lvlib_Process/Initialize.vi", path "C:/Users/XEnderMD/Desktop/CD Project Tools/Built/TimingDRV/Pharlap/TimingDRV Engine.lvlib_Process/Main.vi", path "C:/Users/XEnderMD/Desktop/CD Project Tools/Built/TimingDRV/Pharlap/TimingDRV Engine.lvlib_Assembler/Shutdown.vi", path "C:/Users/XEnderMD/Desktop/CD Project Tools/Built/TimingDRV/Pharlap/TimingDRV Engine.lvlib_Process/Shutdown.vi", path "C:/Users/XEnderMD/Desktop/CD Project Tools/Built/TimingDRV/Engine Release_depinstr.bin"], [path "C:/Users/XEnderMD/Desktop/CD Project Tools/Built/TimingDRV/VxWorks/TimingDRV Engine VxWorks.llb", path "C:/Users/XEnderMD/Desktop/CD Project Tools/Built/TimingDRV/VxWorks/TimingDRV Engine.lvlib_Assembler/Main.vi", path "C:/Users/XEnderMD/Desktop/CD Project Tools/Built/TimingDRV/VxWorks/TimingDRV Engine.lvlib_Input Process/Main.vi", path "C:/Users/XEnderMD/Desktop/CD Project Tools/Built/TimingDRV/VxWorks/TimingDRV Engine.lvlib_Output Process/Initialize Output Channel Values.vi", path "C:/Users/XEnderMD/Desktop/CD Project Tools/Built/TimingDRV/VxWorks/TimingDRV Engine.lvlib_Sine Process/Initialize Output Channel Values.vi", path "C:/Users/XEnderMD/Desktop/CD Project Tools/Built/TimingDRV/VxWorks/TimingDRV Engine.lvlib_Output Process/Update Channel Value.vi", path "C:/Users/XEnderMD/Desktop/CD Project Tools/Built/TimingDRV/VxWorks/TimingDRV Engine.lvlib_Sine Process/Update Channel Value.vi", path "C:/Users/XEnderMD/Desktop/CD Project Tools/Built/TimingDRV/VxWorks/TimingDRV Engine.lvlib_Random Process/Initialize Output Channel Values.vi", path "C:/Users/XEnderMD/Desktop/CD Project Tools/Built/TimingDRV/VxWorks/TimingDRV Engine.lvlib_Random Process/Update Channel Value.vi", path "C:/Users/XEnderMD/Desktop/CD Project Tools/Built/TimingDRV/VxWorks/TimingDRV Engine.lvlib_Assembler/Configure.vi", path "C:/Users/XEnderMD/Desktop/CD Project Tools/Built/TimingDRV/VxWorks/TimingDRV Engine.lvlib_Output Process/Configure.vi", path "C:/Users/XEnderMD/Desktop/CD Project Tools/Built/TimingDRV/VxWorks/TimingDRV Engine.lvlib_Assembler/Initialize.vi", path "C:/Users/XEnderMD/Desktop/CD Project Tools/Built/TimingDRV/VxWorks/TimingDRV Engine.lvlib_Output Process/Initialize.vi", path "C:/Users/XEnderMD/Desktop/CD Project Tools/Built/TimingDRV/VxWorks/TimingDRV Engine.lvlib_Output Process/Main.vi", path "C:/Users/XEnderMD/Desktop/CD Project Tools/Built/TimingDRV/VxWorks/TimingDRV Engine.lvlib_Output Process/Get Output Channel Values.vi", path "C:/Users/XEnderMD/Desktop/CD Project Tools/Built/TimingDRV/VxWorks/TimingDRV Engine.lvlib_Sine Process/Get Output Channel Values.vi", path "C:/Users/XEnderMD/Desktop/CD Project Tools/Built/TimingDRV/VxWorks/TimingDRV Engine.lvlib_Output Process/Set Output Channel Values.vi", path "C:/Users/XEnderMD/Desktop/CD Project Tools/Built/TimingDRV/VxWorks/TimingDRV Engine.lvlib_Sine Process/Set Output Channel Values.vi", path "C:/Users/XEnderMD/Desktop/CD Project Tools/Built/TimingDRV/VxWorks/TimingDRV Engine.lvlib_Output Process/Get Output FIFOs.vi", path "C:/Users/XEnderMD/Desktop/CD Project Tools/Built/TimingDRV/VxWorks/TimingDRV Engine.lvlib_Sine Process/Get Output FIFOs.vi", path "C:/Users/XEnderMD/Desktop/CD Project Tools/Built/TimingDRV/VxWorks/TimingDRV Engine.lvlib_Output Process/Set Output FIFOs.vi", path "C:/Users/XEnderMD/Desktop/CD Project Tools/Built/TimingDRV/VxWorks/TimingDRV Engine.lvlib_Sine Process/Set Output FIFOs.vi", path "C:/Users/XEnderMD/Desktop/CD Project Tools/Built/TimingDRV/VxWorks/TimingDRV Engine.lvlib_Sine Process/Configure.vi", path "C:/Users/XEnderMD/Desktop/CD Project Tools/Built/TimingDRV/VxWorks/TimingDRV Engine.lvlib_Sine Process/Initialize.vi", path "C:/Users/XEnderMD/Desktop/CD Project Tools/Built/TimingDRV/VxWorks/TimingDRV Engine.lvlib_Sine Process/Main.vi", path "C:/Users/XEnderMD/Desktop/CD Project Tools/Built/TimingDRV/VxWorks/TimingDRV Engine.lvlib_Random Process/Get Output Channel Values.vi", path "C:/Users/XEnderMD/Desktop/CD Project Tools/Built/TimingDRV/VxWorks/TimingDRV Engine.lvlib_Random Process/Set Output Channel Values.vi", path "C:/Users/XEnderMD/Desktop/CD Project Tools/Built/TimingDRV/VxWorks/TimingDRV Engine.lvlib_Random Process/Get Output FIFOs.vi", path "C:/Users/XEnderMD/Desktop/CD Project Tools/Built/TimingDRV/VxWorks/TimingDRV Engine.lvlib_Random Process/Set Output FIFOs.vi", path "C:/Users/XEnderMD/Desktop/CD Project Tools/Built/TimingDRV/VxWorks/TimingDRV Engine.lvlib_Random Process/Configure.vi", path "C:/Users/XEnderMD/Desktop/CD Project Tools/Built/TimingDRV/VxWorks/TimingDRV Engine.lvlib_Random Process/Initialize.vi", path "C:/Users/XEnderMD/Desktop/CD Project Tools/Built/TimingDRV/VxWorks/TimingDRV Engine.lvlib_Random Process/Main.vi", path "C:/Users/XEnderMD/Desktop/CD Project Tools/Built/TimingDRV/VxWorks/TimingDRV Engine.lvlib_Process/Configure.vi", path "C:/Users/XEnderMD/Desktop/CD Project Tools/Built/TimingDRV/VxWorks/TimingDRV Engine.lvlib_Assembler/Launcher.vi", path "C:/Users/XEnderMD/Desktop/CD Project Tools/Built/TimingDRV/VxWorks/TimingDRV Engine.lvlib_Process/Launcher.vi", path "C:/Users/XEnderMD/Desktop/CD Project Tools/Built/TimingDRV/VxWorks/TimingDRV Engine.lvlib_Process/Initialize.vi", path "C:/Users/XEnderMD/Desktop/CD Project Tools/Built/TimingDRV/VxWorks/TimingDRV Engine.lvlib_Process/Main.vi", path "C:/Users/XEnderMD/Desktop/CD Project Tools/Built/TimingDRV/VxWorks/TimingDRV Engine.lvlib_Assembler/Shutdown.vi", path "C:/Users/XEnderMD/Desktop/CD Project Tools/Built/TimingDRV/VxWorks/TimingDRV Engine.lvlib_Process/Shutdown.vi", path "C:/Users/XEnderMD/Desktop/CD Project Tools/Built/TimingDRV/Engine Release_depinstr.bin"], [path "C:/Users/XEnderMD/Desktop/CD Project Tools/Built/TimingDRV/Linux_32_ARM/TimingDRV Engine LinuxARM.llb", path "C:/Users/XEnderMD/Desktop/CD Project Tools/Built/TimingDRV/Linux_32_ARM/TimingDRV Engine.lvlib_Assembler/Main.vi", path "C:/Users/XEnderMD/Desktop/CD Project Tools/Built/TimingDRV/Linux_32_ARM/TimingDRV Engine.lvlib_Input Process/Main.vi", path "C:/Users/XEnderMD/Desktop/CD Project Tools/Built/TimingDRV/Linux_32_ARM/TimingDRV Engine.lvlib_Output Process/Initialize Output Channel Values.vi", path "C:/Users/XEnderMD/Desktop/CD Project Tools/Built/TimingDRV/Linux_32_ARM/TimingDRV Engine.lvlib_Sine Process/Initialize Output Channel Values.vi", path "C:/Users/XEnderMD/Desktop/CD Project Tools/Built/TimingDRV/Linux_32_ARM/TimingDRV Engine.lvlib_Output Process/Update Channel Value.vi", path "C:/Users/XEnderMD/Desktop/CD Project Tools/Built/TimingDRV/Linux_32_ARM/TimingDRV Engine.lvlib_Sine Process/Update Channel Value.vi", path "C:/Users/XEnderMD/Desktop/CD Project Tools/Built/TimingDRV/Linux_32_ARM/TimingDRV Engine.lvlib_Random Process/Initialize Output Channel Values.vi", path "C:/Users/XEnderMD/Desktop/CD Project Tools/Built/TimingDRV/Linux_32_ARM/TimingDRV Engine.lvlib_Random Process/Update Channel Value.vi", path "C:/Users/XEnderMD/Desktop/CD Project Tools/Built/TimingDRV/Linux_32_ARM/TimingDRV Engine.lvlib_Assembler/Configure.vi", path "C:/Users/XEnderMD/Desktop/CD Project Tools/Built/TimingDRV/Linux_32_ARM/TimingDRV Engine.lvlib_Output Process/Configure.vi", path "C:/Users/XEnderMD/Desktop/CD Project Tools/Built/TimingDRV/Linux_32_ARM/TimingDRV Engine.lvlib_Assembler/Initialize.vi", path "C:/Users/XEnderMD/Desktop/CD Project Tools/Built/TimingDRV/Linux_32_ARM/TimingDRV Engine.lvlib_Output Process/Initialize.vi", path "C:/Users/XEnderMD/Desktop/CD Project Tools/Built/TimingDRV/Linux_32_ARM/TimingDRV Engine.lvlib_Output Process/Main.vi", path "C:/Users/XEnderMD/Desktop/CD Project Tools/Built/TimingDRV/Linux_32_ARM/TimingDRV Engine.lvlib_Output Process/Get Output Channel Values.vi", path "C:/Users/XEnderMD/Desktop/CD Project Tools/Built/TimingDRV/Linux_32_ARM/TimingDRV Engine.lvlib_Sine Process/Get Output Channel Values.vi", path "C:/Users/XEnderMD/Desktop/CD Project Tools/Built/TimingDRV/Linux_32_ARM/TimingDRV Engine.lvlib_Output Process/Set Output Channel Values.vi", path "C:/Users/XEnderMD/Desktop/CD Project Tools/Built/TimingDRV/Linux_32_ARM/TimingDRV Engine.lvlib_Sine Process/Set Output Channel Values.vi", path "C:/Users/XEnderMD/Desktop/CD Project Tools/Built/TimingDRV/Linux_32_ARM/TimingDRV Engine.lvlib_Output Process/Get Output FIFOs.vi", path "C:/Users/XEnderMD/Desktop/CD Project Tools/Built/TimingDRV/Linux_32_ARM/TimingDRV Engine.lvlib_Sine Process/Get Output FIFOs.vi", path "C:/Users/XEnderMD/Desktop/CD Project Tools/Built/TimingDRV/Linux_32_ARM/TimingDRV Engine.lvlib_Output Process/Set Output FIFOs.vi", path "C:/Users/XEnderMD/Desktop/CD Project Tools/Built/TimingDRV/Linux_32_ARM/TimingDRV Engine.lvlib_Sine Process/Set Output FIFOs.vi", path "C:/Users/XEnderMD/Desktop/CD Project Tools/Built/TimingDRV/Linux_32_ARM/TimingDRV Engine.lvlib_Sine Process/Configure.vi", path "C:/Users/XEnderMD/Desktop/CD Project Tools/Built/TimingDRV/Linux_32_ARM/TimingDRV Engine.lvlib_Sine Process/Initialize.vi", path "C:/Users/XEnderMD/Desktop/CD Project Tools/Built/TimingDRV/Linux_32_ARM/TimingDRV Engine.lvlib_Sine Process/Main.vi", path "C:/Users/XEnderMD/Desktop/CD Project Tools/Built/TimingDRV/Linux_32_ARM/TimingDRV Engine.lvlib_Random Process/Get Output Channel Values.vi", path "C:/Users/XEnderMD/Desktop/CD Project Tools/Built/TimingDRV/Linux_32_ARM/TimingDRV Engine.lvlib_Random Process/Set Output Channel Values.vi", path "C:/Users/XEnderMD/Desktop/CD Project Tools/Built/TimingDRV/Linux_32_ARM/TimingDRV Engine.lvlib_Random Process/Get Output FIFOs.vi", path "C:/Users/XEnderMD/Desktop/CD Project Tools/Built/TimingDRV/Linux_32_ARM/TimingDRV Engine.lvlib_Random Process/Set Output FIFOs.vi", path "C:/Users/XEnderMD/Desktop/CD Project Tools/Built/TimingDRV/Linux_32_ARM/TimingDRV Engine.lvlib_Random Process/Configure.vi", path "C:/Users/XEnderMD/Desktop/CD Project Tools/Built/TimingDRV/Linux_32_ARM/TimingDRV Engine.lvlib_Random Process/Initialize.vi", path "C:/Users/XEnderMD/Desktop/CD Project Tools/Built/TimingDRV/Linux_32_ARM/TimingDRV Engine.lvlib_Random Process/Main.vi", path "C:/Users/XEnderMD/Desktop/CD Project Tools/Built/TimingDRV/Linux_32_ARM/TimingDRV Engine.lvlib_Process/Configure.vi", path "C:/Users/XEnderMD/Desktop/CD Project Tools/Built/TimingDRV/Linux_32_ARM/TimingDRV Engine.lvlib_Assembler/Launcher.vi", path "C:/Users/XEnderMD/Desktop/CD Project Tools/Built/TimingDRV/Linux_32_ARM/TimingDRV Engine.lvlib_Process/Launcher.vi", path "C:/Users/XEnderMD/Desktop/CD Project Tools/Built/TimingDRV/Linux_32_ARM/TimingDRV Engine.lvlib_Process/Initialize.vi", path "C:/Users/XEnderMD/Desktop/CD Project Tools/Built/TimingDRV/Linux_32_ARM/TimingDRV Engine.lvlib_Process/Main.vi", path "C:/Users/XEnderMD/Desktop/CD Project Tools/Built/TimingDRV/Linux_32_ARM/TimingDRV Engine.lvlib_Assembler/Shutdown.vi", path "C:/Users/XEnderMD/Desktop/CD Project Tools/Built/TimingDRV/Linux_32_ARM/TimingDRV Engine.lvlib_Process/Shutdown.vi", path "C:/Users/XEnderMD/Desktop/CD Project Tools/Built/TimingDRV/Engine Release_depinstr.bin"], [path "C:/Users/XEnderMD/Desktop/CD Project Tools/Built/TimingDRV/Linux_x64/TimingDRV Engine Linux64.llb", path "C:/Users/XEnderMD/Desktop/CD Project Tools/Built/TimingDRV/Linux_x64/TimingDRV Engine.lvlib_Assembler/Main.vi", path "C:/Users/XEnderMD/Desktop/CD Project Tools/Built/TimingDRV/Linux_x64/TimingDRV Engine.lvlib_Input Process/Main.vi", path "C:/Users/XEnderMD/Desktop/CD Project Tools/Built/TimingDRV/Linux_x64/TimingDRV Engine.lvlib_Output Process/Initialize Output Channel Values.vi", path "C:/Users/XEnderMD/Desktop/CD Project Tools/Built/TimingDRV/Linux_x64/TimingDRV Engine.lvlib_Sine Process/Initialize Output Channel Values.vi", path "C:/Users/XEnderMD/Desktop/CD Project Tools/Built/TimingDRV/Linux_x64/TimingDRV Engine.lvlib_Output Process/Update Channel Value.vi", path "C:/Users/XEnderMD/Desktop/CD Project Tools/Built/TimingDRV/Linux_x64/TimingDRV Engine.lvlib_Sine Process/Update Channel Value.vi", path "C:/Users/XEnderMD/Desktop/CD Project Tools/Built/TimingDRV/Linux_x64/TimingDRV Engine.lvlib_Random Process/Initialize Output Channel Values.vi", path "C:/Users/XEnderMD/Desktop/CD Project Tools/Built/TimingDRV/Linux_x64/TimingDRV Engine.lvlib_Random Process/Update Channel Value.vi", path "C:/Users/XEnderMD/Desktop/CD Project Tools/Built/TimingDRV/Linux_x64/TimingDRV Engine.lvlib_Assembler/Configure.vi", path "C:/Users/XEnderMD/Desktop/CD Project Tools/Built/TimingDRV/Linux_x64/TimingDRV Engine.lvlib_Output Process/Configure.vi", path "C:/Users/XEnderMD/Desktop/CD Project Tools/Built/TimingDRV/Linux_x64/TimingDRV Engine.lvlib_Assembler/Initialize.vi", path "C:/Users/XEnderMD/Desktop/CD Project Tools/Built/TimingDRV/Linux_x64/TimingDRV Engine.lvlib_Output Process/Initialize.vi", path "C:/Users/XEnderMD/Desktop/CD Project Tools/Built/TimingDRV/Linux_x64/TimingDRV Engine.lvlib_Output Process/Main.vi", path "C:/Users/XEnderMD/Desktop/CD Project Tools/Built/TimingDRV/Linux_x64/TimingDRV Engine.lvlib_Output Process/Get Output Channel Values.vi", path "C:/Users/XEnderMD/Desktop/CD Project Tools/Built/TimingDRV/Linux_x64/TimingDRV Engine.lvlib_Sine Process/Get Output Channel Values.vi", path "C:/Users/XEnderMD/Desktop/CD Project Tools/Built/TimingDRV/Linux_x64/TimingDRV Engine.lvlib_Output Process/Set Output Channel Values.vi", path "C:/Users/XEnderMD/Desktop/CD Project Tools/Built/TimingDRV/Linux_x64/TimingDRV Engine.lvlib_Sine Process/Set Output Channel Values.vi", path "C:/Users/XEnderMD/Desktop/CD Project Tools/Built/TimingDRV/Linux_x64/TimingDRV Engine.lvlib_Output Process/Get Output FIFOs.vi", path "C:/Users/XEnderMD/Desktop/CD Project Tools/Built/TimingDRV/Linux_x64/TimingDRV Engine.lvlib_Sine Process/Get Output FIFOs.vi", path "C:/Users/XEnderMD/Desktop/CD Project Tools/Built/TimingDRV/Linux_x64/TimingDRV Engine.lvlib_Output Process/Set Output FIFOs.vi", path "C:/Users/XEnderMD/Desktop/CD Project Tools/Built/TimingDRV/Linux_x64/TimingDRV Engine.lvlib_Sine Process/Set Output FIFOs.vi", path "C:/Users/XEnderMD/Desktop/CD Project Tools/Built/TimingDRV/Linux_x64/TimingDRV Engine.lvlib_Sine Process/Configure.vi", path "C:/Users/XEnderMD/Desktop/CD Project Tools/Built/TimingDRV/Linux_x64/TimingDRV Engine.lvlib_Sine Process/Initialize.vi", path "C:/Users/XEnderMD/Desktop/CD Project Tools/Built/TimingDRV/Linux_x64/TimingDRV Engine.lvlib_Sine Process/Main.vi", path "C:/Users/XEnderMD/Desktop/CD Project Tools/Built/TimingDRV/Linux_x64/TimingDRV Engine.lvlib_Random Process/Get Output Channel Values.vi", path "C:/Users/XEnderMD/Desktop/CD Project Tools/Built/TimingDRV/Linux_x64/TimingDRV Engine.lvlib_Random Process/Set Output Channel Values.vi", path "C:/Users/XEnderMD/Desktop/CD Project Tools/Built/TimingDRV/Linux_x64/TimingDRV Engine.lvlib_Random Process/Get Output FIFOs.vi", path "C:/Users/XEnderMD/Desktop/CD Project Tools/Built/TimingDRV/Linux_x64/TimingDRV Engine.lvlib_Random Process/Set Output FIFOs.vi", path "C:/Users/XEnderMD/Desktop/CD Project Tools/Built/TimingDRV/Linux_x64/TimingDRV Engine.lvlib_Random Process/Configure.vi", path "C:/Users/XEnderMD/Desktop/CD Project Tools/Built/TimingDRV/Linux_x64/TimingDRV Engine.lvlib_Random Process/Initialize.vi", path "C:/Users/XEnderMD/Desktop/CD Project Tools/Built/TimingDRV/Linux_x64/TimingDRV Engine.lvlib_Random Process/Main.vi", path "C:/Users/XEnderMD/Desktop/CD Project Tools/Built/TimingDRV/Linux_x64/TimingDRV Engine.lvlib_Process/Configure.vi", path "C:/Users/XEnderMD/Desktop/CD Project Tools/Built/TimingDRV/Linux_x64/TimingDRV Engine.lvlib_Assembler/Launcher.vi", path "C:/Users/XEnderMD/Desktop/CD Project Tools/Built/TimingDRV/Linux_x64/TimingDRV Engine.lvlib_Process/Launcher.vi", path "C:/Users/XEnderMD/Desktop/CD Project Tools/Built/TimingDRV/Linux_x64/TimingDRV Engine.lvlib_Process/Initialize.vi", path "C:/Users/XEnderMD/Desktop/CD Project Tools/Built/TimingDRV/Linux_x64/TimingDRV Engine.lvlib_Process/Main.vi", path "C:/Users/XEnderMD/Desktop/CD Project Tools/Built/TimingDRV/Linux_x64/TimingDRV Engine.lvlib_Assembler/Shutdown.vi", path "C:/Users/XEnderMD/Desktop/CD Project Tools/Built/TimingDRV/Linux_x64/TimingDRV Engine.lvlib_Process/Shutdown.vi", path "C:/Users/XEnderMD/Desktop/CD Project Tools/Built/TimingDRV/Engine Release_depinstr.bin"]] ("Generated files 2"), "Project XML Editor in"=w9) -> ("error out"=w8:errorcluster, "Dependency Parameters"=w6:T1[], "Project XML Editor out"=w7:refnum<class "Project XML Editor.lvclass">)  [unwired: 6 in]
      "Array" <- w6
      n5 = for {
        shift-right: [w19] -> w13
        shift-left: w8 -> [w18]
        shift-right: [w20] -> w14
        shift-left: w7 -> [w17]
        tunnel: w6 -> [w16] mode=indexing
        n6 = call "Add XML Dependency.vi"("error in (no error)"=w18, "Dependency Parameters"=w16, "Project XML Editor in"=w17) -> ("error out"=w19:errorcluster, "Project XML Editor out"=w20:refnum<class "Project XML Editor.lvclass">)  [unwired: 7 in]
      }
    }
    frame Enabled {
      n7 = call "Get CD Name.vi"("Project XML Editor in"=w26) -> ("CD Name"=→"CD Name":string, "Project XML Editor out"=w22:refnum<class "Project XML Editor.lvclass">)  [unwired: 9 in]
      n8 = call "Get Common Doc Dir.vi"("Project XML Editor in"=w22) -> ("Common Doc Dir"=→"Common Doc Dir":string)  [unwired: 9 in, 1 out]
      n9 = call "Get XML Path.vi"("Project XML Editor in"=w22) -> ("XML Path"=→"XML Path":path)  [unwired: 9 in, 1 out]
    }
  }
  n10 = call "Destroy XML Editor.vi"("error in (no error)"=w3, "Project XML Editor in"=w4) -> ("error out"=→"error out":errorcluster)  [unwired: 9 in]
